vi "cursor.vi"(10 "Bpm":i32[](array[numeric]), 11 "CrsrList in":T1) -> (3 "CrsrList out":T1)   [LabVIEW 2024]
uses:
  <vilib>/Utility/miscctls.llb/LVCursorListTypeDef.ctl
  <vilib>/Analysis/baseanly.llb/Mean (DBL).vi
  <vilib>/Analysis/NI_AALBase.lvlib
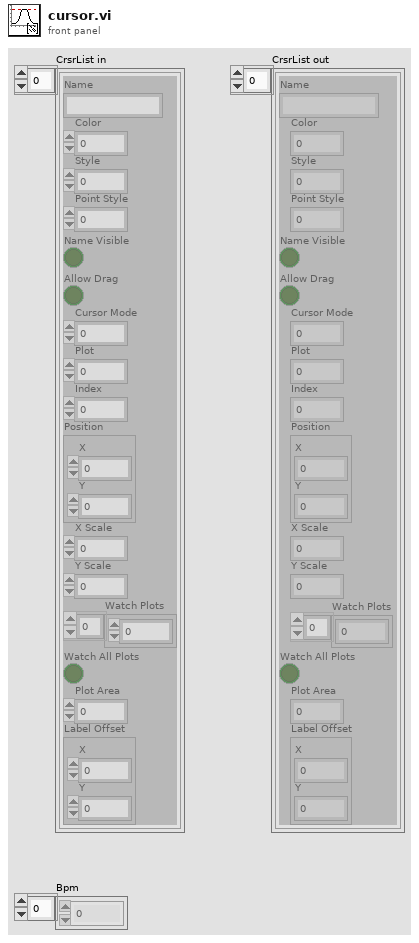
[diagram p1: front panel]
types:
  T1 = typedef "LVCursorListTypeDef.ctl" = cluster{"Name":string, "Color":u32, "Style":u8, "Point Style":u8, "Name Visible":bool, "Allow Drag":bool, "Cursor Mode":u32, "Plot":i32, "Index":i32, "Position":cluster{"X":dbl, "Y":dbl}, "X Scale":u32, "Y Scale":u32, "Watch Plots":i32[], "Watch All Plots":bool, "Plot Area":i32, "Label Offset":cluster{"X":dbl, "Y":dbl}}[]
  T2 = cluster{"Name":string, "Color":u32, "Style":u8, "Point Style":u8, "Name Visible":bool, "Allow Drag":bool, "Cursor Mode":u32, "Plot":i32, "Index":i32, "Position":cluster{"X":dbl, "Y":dbl}, "X Scale":u32, "Y Scale":u32, "Watch Plots":i32[], "Watch All Plots":bool, "Plot Area":i32, "Label Offset":cluster{"X":dbl, "Y":dbl}}
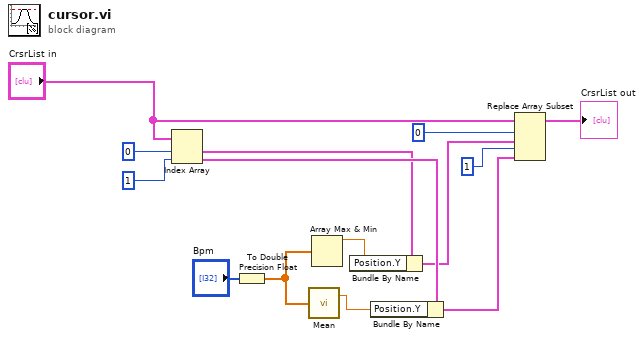
[diagram p0: block diagram]
diagram:
  n1 = Index Array(array="CrsrList in", index #1=0 ("index"), index #2=1 ("index")) -> (element #1=w7:T2, element #2=w8:T2)
  n2 = To Double Precision Float(number="Bpm") -> (double precision float=w14:dbl[])
  n3 = call-poly <vilib>:"Mean.vi"("X"=w14) -> ("mean"=w4:dbl)  [unwired: 1 out]
  n4 = Array Max & Min(array=w14) -> (max value=w2:dbl)  [unwired: 3 out]
  n5 = Bundle By Name(cluster=w7, "Position.Y"=w2) -> (w6:T2)
  n6 = Bundle By Name(cluster=w8, "Position.Y"=w4) -> (w5:T2)
  n7 = Replace Array Subset(array="CrsrList in", new element #1=w6, index #1=0 ("index"), new element #2=w5, index #2=1 ("index")) -> (→"CrsrList out":T1)
